vi "test-swerve-drive-kinematics-09.vi"() -> (3 "Test Passed":bool)   [LabVIEW 2019]
uses:
  <vilib>/Rock Robotics/WPI/ThirdParty/JAS_Junk/TrajLib/SWERVE_DRIVE_MODULE_STATE.ctl
  <vilib>/Rock Robotics/WPI/ThirdParty/JAS_Junk/TrajLib/ROTATION2D.ctl
  <vilib>/Rock Robotics/WPI/ThirdParty/JAS_Junk/TrajLib/Rotation_CreateAngle.vi
  <vilib>/Rock Robotics/WPI/ThirdParty/JAS_Junk/TrajLib/Trajectory_Library.lvlib
panel:
  out "ModuleStates":T1[](array[typedef]) {"Angle"."SIN" format="%13.4f"; "Angle"."COS" format="%13.4f"; "Angle"."VALUE" format="%13.4f"}
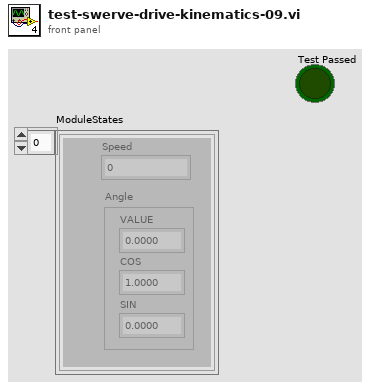
[diagram p1: front panel]
types:
  T1 = typedef "Trajectory_Library.lvlib/SWERVE_DRIVE_MODULE_STATE.ctl" = cluster{"Speed":dbl, "Angle":T2}
  T2 = typedef "Trajectory_Library.lvlib/ROTATION2D.ctl" = cluster{"VALUE":dbl, "COS":dbl, "SIN":dbl}
  T3 = typedef "Trajectory_Library.lvlib/TRANSLATION2D.ctl" = cluster{"X":dbl, "Y":dbl}
  T4 = typedef "Trajectory_Library.lvlib/SWERVE_DRIVE_KINEMATICS.ctl" = cluster{"NumModules":i32, "InverseKinematics":T5, "ForwardKinematics":T5, "Modules":T3[], "PrevCoR":T3}
  T5 = typedef "NI_Matrix.lvlib/RealMatrix.ctl" = dbl[][]
  T6 = typedef "Trajectory_Library.lvlib/CHASSIS_SPEEDS.ctl" = cluster{"vX":dbl, "vY":dbl, "vOmega":dbl}
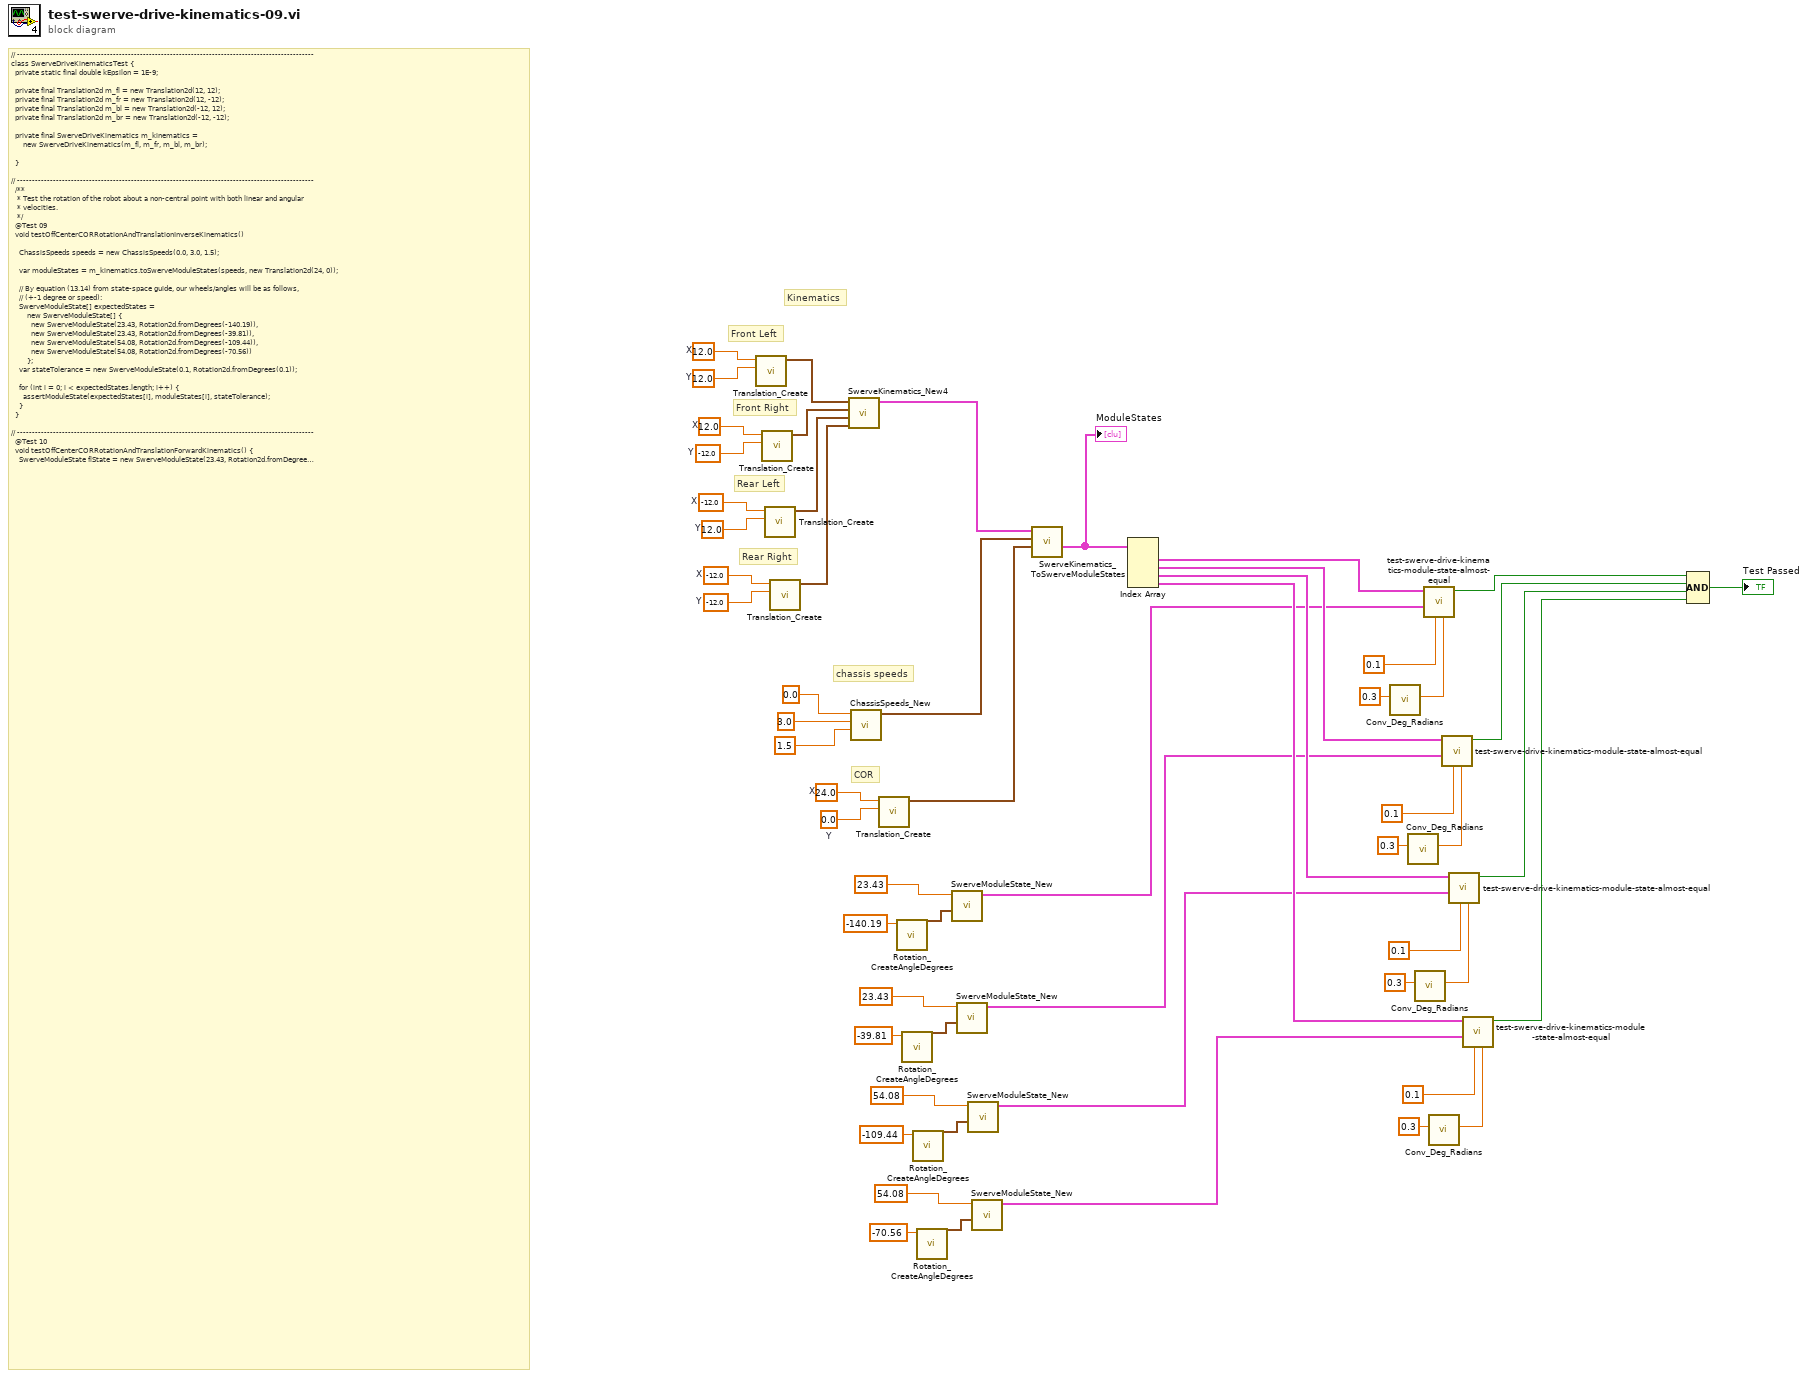
[diagram p0: block diagram]
diagram:
  w39 = 24.0  # X
  w38 = 0.0  # Y
  w53 = -12.0  # X
  w52 = -12.0  # Y
  w51 = -12.0  # X
  w50 = 12.0  # Y
  w49 = 12.0  # X
  w48 = -12.0  # Y
  w47 = 12.0  # X
  w46 = 12.0  # Y
  # "COR"
  # "Kinematics"
  # "Rear Right"
  # "Rear Left"
  # "Front Right"
  # "Front Left"
  # "chassis speeds"
  # "// ---------------------------------------------------------------------------------------------------\nclass SwerveDriveKinematicsTest {\n  private static final double kEpsilon = 1E-9;\n\n  private final Translation2d m_fl = new Translation2d(12, 12);\n  private final Translation2d m_fr = new Translation2d(12, -12);\n  private final Translation2d m_bl = new Translation2d(-12, 12);\n  private final Translation2d m_br = new Translation2d(-12, -12);\n\n  private final SwerveDriveKinematics m_kinematics =\n      new SwerveDriveKinematics(m_fl, m_fr, m_bl, m_br);\n\n  }\n\n// ---------------------------------------------------------------------------------------------------\n  /**\n   * Test the rotation of the robot about a non-central point with both linear and angular\n   * velocities.\n   */\n  @Test 09\n  void testOffCenterCORRotationAndTranslationInverseKinematics() \n\n    ChassisSpeeds speeds = new ChassisSpeeds(0.0, 3.0, 1.5);\n\n    var moduleStates = m_kinematics.toSwerveModuleStates(speeds, new Translation2d(24, 0));\n\n    // By equation (13.14) from state-space guide, our wheels/angles will be as follows,\n    // (+-1 degree or speed):\n    SwerveModuleState[] expectedStates =\n        new SwerveModuleState[] {\n          new SwerveModuleState(23.43, Rotation2d.fromDegrees(-140.19)),\n          new SwerveModuleState(23.43, Rotation2d.fromDegrees(-39.81)),\n          new SwerveModuleState(54.08, Rotation2d.fromDegrees(-109.44)),\n          new SwerveModuleState(54.08, Rotation2d.fromDegrees(-70.56))\n        };\n    var stateTolerance = new SwerveModuleState(0.1, Rotation2d.fromDegrees(0.1));\n\n    for (int i = 0; i < expectedStates.length; i++) {\n      assertModuleState(expectedStates[i], moduleStates[i], stateTolerance);\n    }\n  }\n\n// ---------------------------------------------------------------------------------------------------\n  @Test 10\n  void testOffCenterCORRotationAndTranslationForwardKinematics() {\n    SwerveModuleState flState = new SwerveModuleState(23.43, Rotation2d.fromDegrees(-140.19));\n    SwerveModuleState frState = new SwerveModuleState(23.43, Rotation2d.fromDegrees(-39.81));\n    SwerveModuleState blState = new SwerveModuleState(54.08, Rotation2d.fromDegrees(-109.44));\n    SwerveModuleState brState = new SwerveModuleState(54.08, Rotation2d.fromDegrees(-70.56));\n\n    var chassisSpeeds = m_kinematics.toChassisSpeeds(flState, frState, blState, brState);\n\n    /*\n    From equation (13.17), we know that chassis motion is th dot product of the\n    pseudoinverse of the inverseKinematics matrix (with the center of rotation at\n    (0,0) -- we don't want the motion of the center of rotation, we want it of\n    the center of the robot). These above SwerveModuleStates are known to be from\n    a velocity of [[0][3][1.5]] about (0, 24), and the expected numbers have been\n    calculated using Numpy's linalg.pinv function.\n    */\n\n    assertAll(\n        () -> assertEquals(0.0, chassisSpeeds.vxMetersPerSecond, 0.1),\n        () -> assertEquals(-33.0, chassisSpeeds.vyMetersPerSecond, 0.1),\n        () -> assertEquals(1.5, chassisSpeeds.omegaRadiansPerSecond, 0.1));\n  }\n\n// ---------------------------------------------------------------------------------------------------\n  @Test 11\n  void testNormalize() {\n    SwerveModuleState fl = new SwerveModuleState(5, new Rotation2d());\n    SwerveModuleState fr = new SwerveModuleState(6, new Rotation2d());\n    SwerveModuleState bl = new SwerveModuleState(4, new Rotation2d());\n    SwerveModuleState br = new SwerveModuleState(7, new Rotation2d());\n\n    SwerveModuleState[] arr = {fl, fr, bl, br};\n    SwerveDriveKinematics.normalizeWheelSpeeds(arr, 5.5);\n\n    double factor = 5.5 / 7.0;\n\n    assertAll(\n        () -> assertEquals(5.0 * factor, arr[0].speedMetersPerSecond, kEpsilon),\n        () -> assertEquals(6.0 * factor, arr[1].speedMetersPerSecond, kEpsilon),\n        () -> assertEquals(4.0 * factor, arr[2].speedMetersPerSecond, kEpsilon),\n        () -> assertEquals(7.0 * factor, arr[3].speedMetersPerSecond, kEpsilon));\n  }\n}"
  n1 = call <vilib>:"Translation_Create.vi"("Y"=w46, "X"=w47) -> ("TRANSLATION"=w41:T3)  [unwired: 9 in]
  n2 = call <vilib>:"Translation_Create.vi"("Y"=w48, "X"=w49) -> ("TRANSLATION"=w54:T3)  [unwired: 9 in]
  n3 = call <vilib>:"Translation_Create.vi"("Y"=w50, "X"=w51) -> ("TRANSLATION"=w55:T3)  [unwired: 9 in]
  n4 = call <vilib>:"Translation_Create.vi"("Y"=w52, "X"=w53) -> ("TRANSLATION"=w56:T3)  [unwired: 9 in]
  n5 = call <vilib>:"SwerveKinematics_New4.vi"("wheel 3"=w56, "wheel 2"=w55, "wheel 1"=w54, "wheel 0"=w41) -> ("SWERVE_DRIVE_KINEMATICS"=w45:T4)  [unwired: 7 in]
  n6 = call <vilib>:"ChassisSpeeds_New.vi"("vAngular"=1.5, "vY"=3.0, "vX"=0.0) -> ("CHASSIS"=w44:T6)  [unwired: 8 in]
  n7 = call <vilib>:"Translation_Create.vi"("Y"=w38, "X"=w39) -> ("TRANSLATION"=w37:T3)  [unwired: 9 in]
  n8 = call <vilib>:"Rotation_CreateAngleDegrees.vi"("Angle_Degrees"=-140.19) -> ("ROTATION"=w36:T2)  [unwired: 10 in]
  n9 = call <vilib>:"Rotation_CreateAngleDegrees.vi"("Angle_Degrees"=-39.81) -> ("ROTATION"=w33:T2)  [unwired: 10 in]
  n10 = call <vilib>:"Rotation_CreateAngleDegrees.vi"("Angle_Degrees"=-109.44) -> ("ROTATION"=w30:T2)  [unwired: 10 in]
  n11 = call <vilib>:"Rotation_CreateAngleDegrees.vi"("Angle_Degrees"=-70.56) -> ("ROTATION"=w27:T2)  [unwired: 10 in]
  n12 = call <vilib>:"SwerveModuleState_New.vi"("ROTATION"=w36, "Speed"=23.43) -> ("SWERVE_DRIVE_MODULE_STATE"=w8:T1)  [unwired: 9 in]
  n13 = call <vilib>:"SwerveModuleState_New.vi"("ROTATION"=w33, "Speed"=23.43) -> ("SWERVE_DRIVE_MODULE_STATE"=w7:T1)  [unwired: 9 in]
  n14 = call <vilib>:"SwerveModuleState_New.vi"("ROTATION"=w30, "Speed"=54.08) -> ("SWERVE_DRIVE_MODULE_STATE"=w6:T1)  [unwired: 9 in]
  n15 = call <vilib>:"SwerveModuleState_New.vi"("ROTATION"=w27, "Speed"=54.08) -> ("SWERVE_DRIVE_MODULE_STATE"=w5:T1)  [unwired: 9 in]
  n16 = call <vilib>:"SwerveKinematics_ToSwerveModuleStates.vi"("CenterOfRotation"=w37, "ChassisSpeeds"=w44, "in SWERVE_DRIVE_KINEMATICS"=w45) -> ("ModuleStates"=w43:T1[])  [unwired: 7 in, 1 out]
  "ModuleStates" <- w43
  n17 = Index Array(array=w43) -> (element #1=w12:T1, element #2=w11:T1, element #3=w10:T1, element #4=w9:T1)  [unwired: 4 in]
  n18 = call <vilib>:"Conv_Deg_Radians.vi"("Degress"=0.3) -> ("Radians"=w15:dbl)  [unwired: 10 in]
  n19 = call <vilib>:"Conv_Deg_Radians.vi"("Degress"=0.3) -> ("Radians"=w24:dbl)  [unwired: 10 in]
  n20 = call <vilib>:"Conv_Deg_Radians.vi"("Degress"=0.3) -> ("Radians"=w21:dbl)  [unwired: 10 in]
  n21 = call "test-swerve-drive-kinematics-module-state-almost-equal.vi"("Tolerance Deg"=w15, "Tolerance Speed"=0.1, "mod State 1"=w8, "mod State 0"=w12) -> ("Approx Equal"=w4:bool)  [unwired: 7 in]
  n22 = call <vilib>:"Conv_Deg_Radians.vi"("Degress"=0.3) -> ("Radians"=w18:dbl)  [unwired: 10 in]
  n23 = call "test-swerve-drive-kinematics-module-state-almost-equal.vi"("Tolerance Deg"=w24, "Tolerance Speed"=0.1, "mod State 1"=w7, "mod State 0"=w11) -> ("Approx Equal"=w3:bool)  [unwired: 7 in]
  n24 = call "test-swerve-drive-kinematics-module-state-almost-equal.vi"("Tolerance Deg"=w21, "Tolerance Speed"=0.1, "mod State 1"=w6, "mod State 0"=w10) -> ("Approx Equal"=w2:bool)  [unwired: 7 in]
  n25 = call "test-swerve-drive-kinematics-module-state-almost-equal.vi"("Tolerance Deg"=w18, "Tolerance Speed"=0.1, "mod State 1"=w5, "mod State 0"=w9) -> ("Approx Equal"=w1:bool)  [unwired: 7 in]
  n26 = Compound Arithmetic op=AND(w4, w3, w2, w1) -> (→"Test Passed":bool)
